vi "Configure Scaling.vi"(0 "VISA resource name":refnum<visa-resource-name>, 1 "Scaling Constant A (1.0)":dbl=1.0 min=-9.99999e+26 max=9.99999e+26 step=1e-15 format="%_6g", 2 "Scaling Constant C (1.0)":dbl=1.0 min=-9.99999e+26 max=9.99999e+26 step=1e-15 format="%_6g", 5 "Enable Calculate Scaling (F: Disable)":bool, 11 "error in (no error)":errorcluster, 12 "Scaling Constant B (0.0)":dbl min=-9.99999e+26 max=9.99999e+26 step=1e-15 format="%_6g") -> (4 "VISA resource name out":refnum<visa-resource-name>, 15 "error out":errorcluster)   [LabVIEW 2017, in "ADCMT 6240.lvlib"]
doc: "This VI configures the Scaling calculation."
uses:
  ADCMT 6240.lvlib
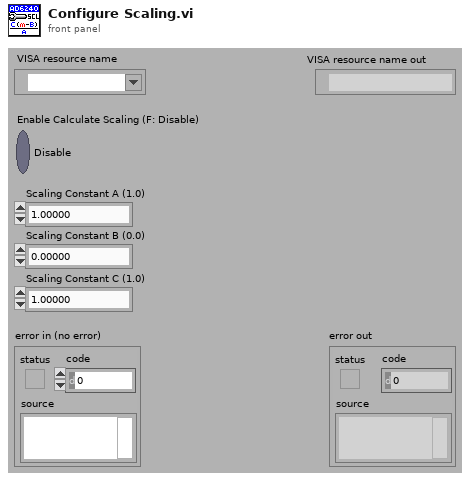
[diagram p1: front panel]
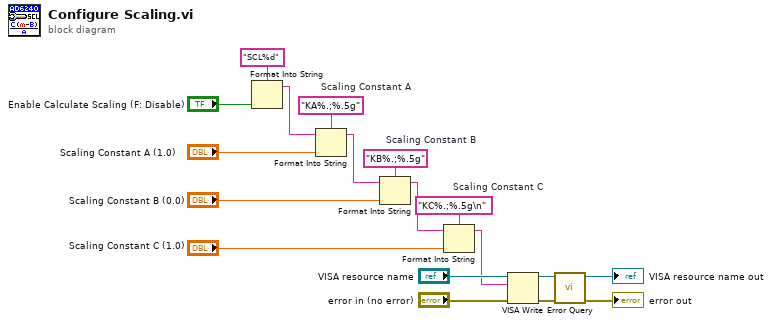
[diagram p0: block diagram]
diagram:
  w8 = "KC%.;%.5g\n"  # Scaling Constant C
  w7 = "KB%.;%.5g"  # Scaling Constant B
  w9 = "KA%.;%.5g"  # Scaling Constant A
  n1 = Format Into String ("文字列にフォーマット")(format string="SCL%d", "Enable Calculate Scaling (F: Disable)") -> (resulting string=w4:string)  [unwired: 2 in, 1 out]
  n2 = Format Into String ("文字列にフォーマット")(format string=w9, initial string=w4, "Scaling Constant A (1.0)") -> (resulting string=w3:string)  [unwired: 1 in, 1 out]
  n3 = Format Into String ("文字列にフォーマット")(format string=w7, initial string=w3, "Scaling Constant B (0.0)") -> (resulting string=w2:string)  [unwired: 1 in, 1 out]
  n4 = Format Into String ("文字列にフォーマット")(format string=w8, initial string=w2, "Scaling Constant C (1.0)") -> (resulting string=w1:string)  [unwired: 1 in, 1 out]
  n5 = VISA Write ("VISA書き込み")(VISA resource name="VISA resource name", write buffer=w1, error in (no error)="error in (no error)") -> (VISA resource name out=w14:refnum<visa-resource-name>, error out=w13:errorcluster)  [unwired: 1 out]
  n6 = call "Error Query.vi"("error in (no error)"=w13, "VISA resource name"=w14) -> ("error out"=→"error out":errorcluster, "VISA resource name out"=→"VISA resource name out":refnum<visa-resource-name>)  [unwired: 6 in, 2 out]
